vi "Graph Get Color List Element.vi"(6 "index":i32, 8 "Error In":errorcluster, 9 "Color":u32(colorbox), 10 "Color List":string(combo), 11 "Color Chooser":enum16{"unchanged", "Color Box", "Color List"}(ring)) -> (0 "Error Out":errorcluster, 1 "Color":u32, 3 "Color defined?":bool)   [LabVIEW 2021, in "Graphs.lvlib"]
uses:
  Graphs.lvlib
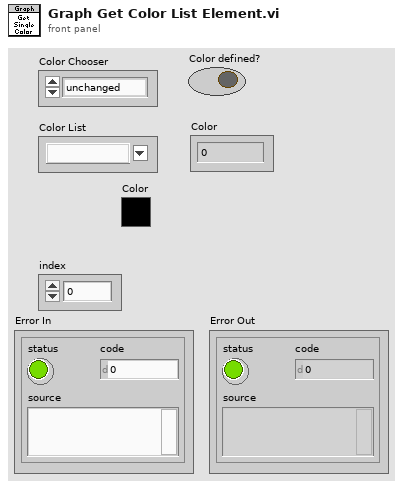
[diagram p1: front panel]
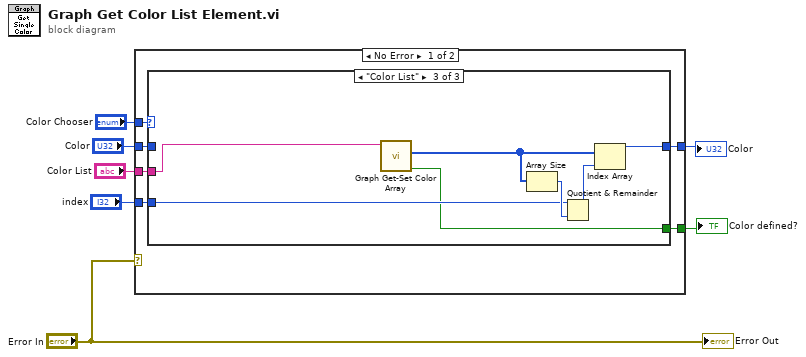
[diagram p0: block diagram]
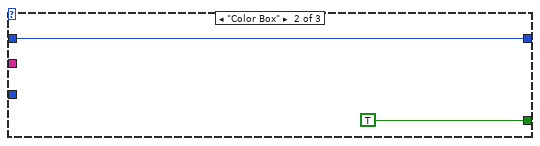
[diagram p3: hidden frame]
diagram:
  n1 = case shown="No Error" "Error In" {
    tunnel: "Color Chooser" -> [w13 _]
    tunnel: "Color" -> [w12 _]
    tunnel: [w11 _] -> w5
    tunnel: [w10 _] -> w4
    tunnel: "Color List" -> [w9 _]
    tunnel: "index" -> [w8 _]
    frame No Error {
      n2 = case shown="\"Color List\"" w13 {
        tunnel: w12 -> [_ w15 _]
        tunnel: [_ w15 w18] -> w11
        tunnel: [_ TRUE ("Color defined?") w17] -> w10
        tunnel: w9 -> [_ _ w22]
        tunnel: w8 -> [_ _ w20]
        frame "unchanged", Default {
        }
        frame "Color Box" {
        }
        frame "Color List" {
          n3 = call "Graph Get-Set Color Array.vi"("Color List Name"=w22) -> ("Found?"=w17:bool, "Color Array (out)"=w16:u32[])  [unwired: 5 in, 4 out]
          n4 = Array Size(array=w16) -> (size(s)=w21:i32)
          n5 = Quotient & Remainder(x=w20, y=w21) -> (x-y*floor(x/y)=w19:i32)  [unwired: 1 out]
          n6 = Index Array(array=w16, index=w19) -> (element=w18:u32)
        }
      }
    }
    frame Error {
    }
  }
  "Color" <- w5
  "Color defined?" <- w4
  "Error Out" <- "Error In"
